vi "TestExeVIPath.vi"() -> ()   [LabVIEW 2016]
panel:
  in  "布尔":bool
  out "VI路径":path
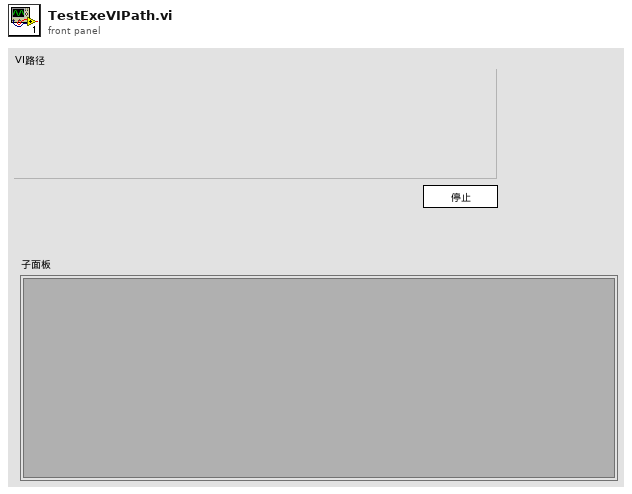
[diagram p1: front panel]
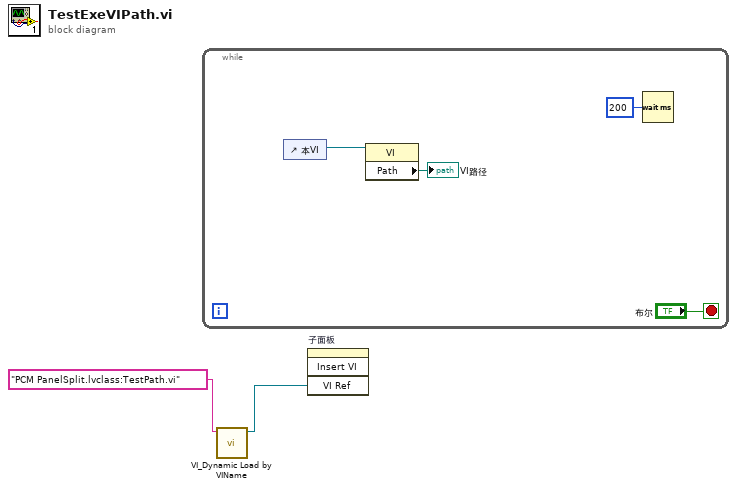
[diagram p0: block diagram]
diagram:
  n1 = while {
    stop <- "布尔" stop-if-true
    n2 = control-ref of="本VI"() -> (w6:refnum<vi>)
    n3 = property class="VI"(reference=w6) -> ("Path"=→"VI路径":path)  [unwired: 1 in, 2 out]
    n4 = Wait (ms)(milliseconds to wait=u32 200 ("等待时间（毫秒）")) -> ()  [unwired: 1 out]
  }
  n5 = call "VI_Dynamic Load by VIName.vi"("VI Name"="PCM PanelSplit.lvclass:TestPath.vi" ("VI名称")) -> ("Dynamic vi reference out"=w2:refnum<vi>)  [unwired: 8 in, 2 out]
  n6 = invoke on="子面板" class="SubPnl" method="Insert VI"("VI Ref"=w2) -> ()  [unwired: 3 in, 4 out]
